vi "new.vi"(11 "timer":i32) -> (3 "wait action out":refnum<class "wait action.lvclass">)   [LabVIEW 2014, in "wait action.lvclass"]
uses:
  wait action.lvclass
  wait action.lvclass/wait action.ctl
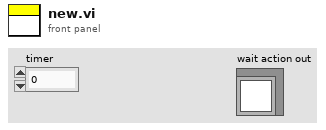
[diagram p1: front panel]
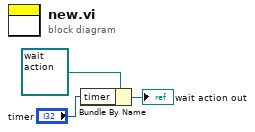
[diagram p0: block diagram]
diagram:
  n1 = Bundle By Name(cluster=refnum<class "wait action.lvclass"> refnum ("wait action in"), "timer"="timer") -> (→"wait action out":refnum<class "wait action.lvclass">)
